vi "Voltage Write Single.vi"(8 "error in":errorcluster, 9 "Channel Index":i32=1, 10 "Voltage AV":dbl, 11 "Power Supply In":refnum<class "Power Supply.lvclass">) -> (0 "error out":errorcluster, 3 "Power Supply Out":refnum<class "Power Supply.lvclass">)   [LabVIEW 2023, in "Power Supply.lvclass"]
uses:
  Power Supply.lvclass
  Power Supply.lvclass/Power Supply.ctl
  Low Level Capabilities/Voltage/Voltage Actual Value/Voltage Actual Value.lvclass
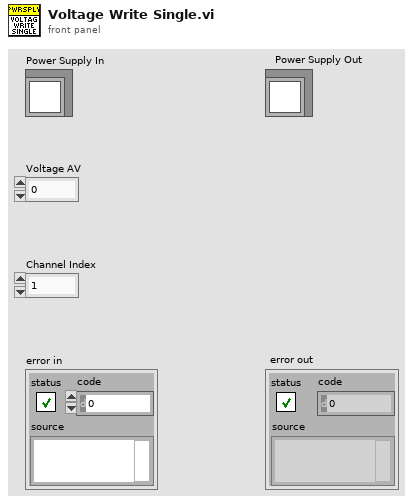
[diagram p1: front panel]
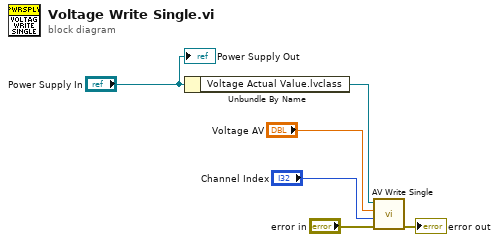
[diagram p0: block diagram]
diagram:
  n1 = Unbundle By Name("Power Supply In") -> ("Voltage Actual Value.lvclass"=w5:refnum<class "Voltage Actual Value.lvclass">)
  n2 = call-dynamic "AV Write Single.vi"("error in"="error in", "Channel Index"="Channel Index", "Voltage AV"="Voltage AV", "Voltage Actual Value in"=w5) -> ("error out"=→"error out":errorcluster)  [unwired: 6 in, 1 out]
  "Power Supply Out" <- "Power Supply In"
